vi "Server_Demo_VIs_ajg.vi"(11 "Only get This VIs path":bool) -> (3 "path":path)   [LabVIEW 2013]
doc: "reentrant"
panel:
  in  "org demo":bool
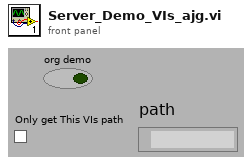
[diagram p1: front panel]
types:
  T1 = typedef "vi picker-ajg.ctl" = enum32{"Choose Something", "QUIT", "M1Cam", "M2Cam", "M4Cam", "M5Cam", "LP_Mode", "M3HPD_CCD_Near", "PhasicsHPD", "TEA_HPLBD_EnergyMeter", "LB_HPBD_EnergyMeter", "OpenHouse Demo", "demo"}
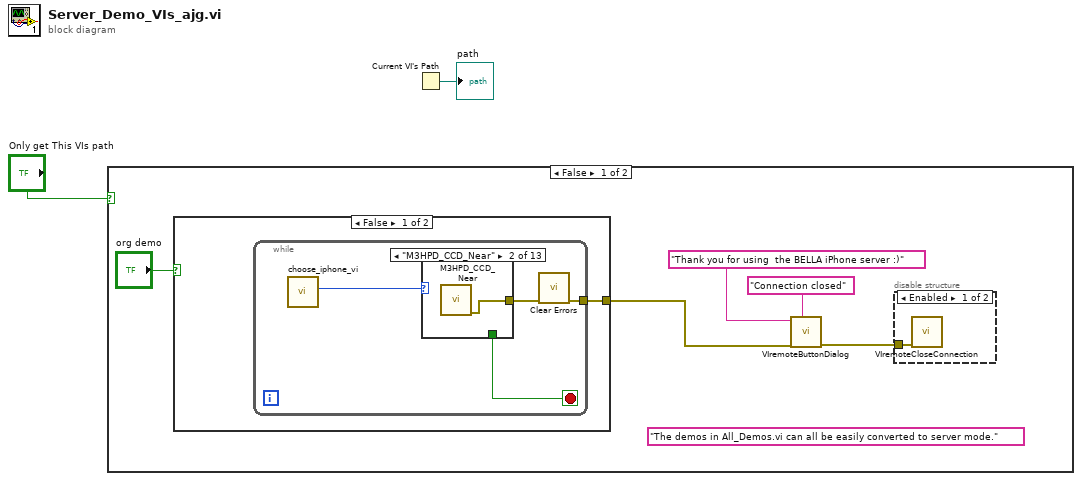
[diagram p0: block diagram]
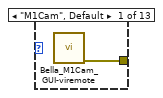
[diagram p3: hidden frame]
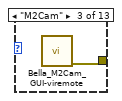
[diagram p4: hidden frame]
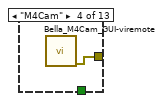
[diagram p5: hidden frame]
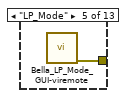
[diagram p6: hidden frame]
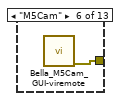
[diagram p7: hidden frame]
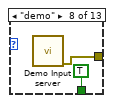
[diagram p9: hidden frame]
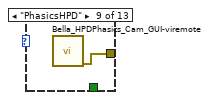
[diagram p10: hidden frame]
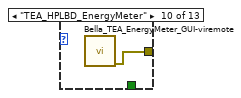
[diagram p11: hidden frame]
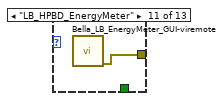
[diagram p12: hidden frame]
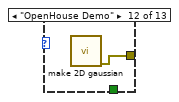
[diagram p13: hidden frame]
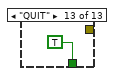
[diagram p14: hidden frame]
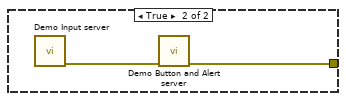
[diagram p15: hidden frame]
diagram:
  n1 = case shown="False" "Only get This VIs path" {
    frame False {
      (unwired) "The demos in All_Demos.vi can all be easily converted to server mode." ("message")
      n2 = case shown="False" "org demo" {
        tunnel: [w9 w27] -> w3
        frame False {
          n3 = while {
            tunnel: [w12] -> w9
            stop <- w10 stop-if-true
            n4 = call "choose_iphone_vi.vi"() -> ("Vi to run ind"=w11:T1)  [unwired: 10 in, 1 out]
            n5 = case shown="\"M3HPD_CCD_Near\"" w11 {
              tunnel: [w14 w15 w16 w17 w18 w19 _ w21 w22 w23 w24 w25 _] -> w13
              tunnel: [_ _ _ _ _ _ _ TRUE _ _ _ _ TRUE] -> w10
              frame "M1Cam", Default {
                n6 = call "Bella_M1Cam_GUI-viremote.vi"() -> ("error IO 2"=w14:errorcluster)  [unwired: 11 in]
              }
              frame "M3HPD_CCD_Near" {
                n7 = call "M3HPD_CCD_Near.vi"() -> ("error IO 2"=w15:errorcluster)  [unwired: 11 in]
              }
              frame "M2Cam" {
                n8 = call "Bella_M2Cam_GUI-viremote.vi"() -> ("error IO 2"=w16:errorcluster)  [unwired: 11 in]
              }
              frame "M4Cam" {
                n9 = call "Bella_M4Cam_GUI-viremote.vi"() -> ("error IO 2"=w17:errorcluster)  [unwired: 11 in]
              }
              frame "LP_Mode" {
                n10 = call "Bella_LP_Mode_GUI-viremote.vi"() -> ("error IO 2"=w18:errorcluster)  [unwired: 11 in]
              }
              frame "M5Cam" {
                n11 = call "Bella_M5Cam_GUI-viremote.vi"() -> ("error IO 2"=w19:errorcluster)  [unwired: 11 in]
              }
              frame "Choose Something" {
              }
              frame "demo" {
                n12 = call "Demo Input server.vi"() -> ("error out"=w21:errorcluster)  [unwired: 10 in, 1 out]
              }
              frame "PhasicsHPD" {
                n13 = call "Bella_HPDPhasics_Cam_GUI-viremote.vi"() -> ("error IO 2"=w22:errorcluster)  [unwired: 11 in]
              }
              frame "TEA_HPLBD_EnergyMeter" {
                n14 = call "Bella_TEA_EnergyMeter_GUI-viremote.vi"() -> ("error IO 2"=w23:errorcluster)  [unwired: 11 in]
              }
              frame "LB_HPBD_EnergyMeter" {
                n15 = call "Bella_LB_EnergyMeter_GUI-viremote.vi"() -> ("error IO 2"=w24:errorcluster)  [unwired: 11 in]
              }
              frame "OpenHouse Demo" {
                n16 = call "make 2D gaussian.vi"() -> ("error out"=w25:errorcluster)  [unwired: 10 in, 1 out]
              }
              frame "QUIT" {
              }
            }
            n17 = call <vilib>:"Clear Errors.vi"("error in (no error)"=w13) -> ("error out"=w12:errorcluster)  [unwired: 6 in]
          }
        }
        frame True {
          n18 = call "Demo Input server.vi"() -> ("error out"=w28:errorcluster)  [unwired: 1 in, 10 out]
          n19 = call "Demo Button and Alert server.vi"("error in (no error)"=w28) -> ("error out"=w27:errorcluster)  [unwired: 10 out]
        }
      }
      n20 = call "VIremoteButtonDialog.vi"("Window Title (\"\")"="Connection closed" ("Window Title (\"\")"), "error in (no error)"=w3, "message"="Thank you for using  the BELLA iPhone server :)") -> ("error out"=w5:errorcluster)  [unwired: 1 in, 7 out]
      n21 = disable-structure shown="Enabled" {
        disable-tunnel: w5 -> [w8 _]
        frame Enabled {
          n22 = call "VIremoteCloseConnection.vi"("error in (no error)"=w8) -> ()  [unwired: 1 in, 10 out]
        }
        frame Disabled {
        }
      }
    }
    frame True {
    }
  }
  n23 = Current VI's Path() -> (path=→"path":path)
